vi "Channel plots.vi"(0 "Current time":timestamp[](array[timestamp]), 1 "In Channels":sgl[][](array[numeric]), 3 "Input Channels":dbl[](array[numeric])=[0.0, 0.0, 0.0, 0.0, 0.0, 0.0, 0.0, 0.0, 0.0, 0.0, 0.0, 0.0]) -> (2 "output graph":T1(array[cluster]), 4 "out Ch 1":dbl[](array[numeric]), 5 "out Ch 6":dbl[](array[numeric]), 6 "out Ch 2":dbl[](array[numeric]), 7 "out Ch 3":dbl[](array[numeric]), 8 "out Ch 4":dbl[](array[numeric]), 9 "out Ch 5":dbl[](array[numeric]))   [LabVIEW 2018]
panel:
  # "Ch 0"
  # "Ch 1"
  # "Ch 2"
  # "Ch 3"
  # "Ch 4"
  # "Ch 5"
  # "Ch 6"
  # "Ch 7"
  # "Ch 8"
  # "Ch 9"
  # "Ch 10"
  # "Ch 11"
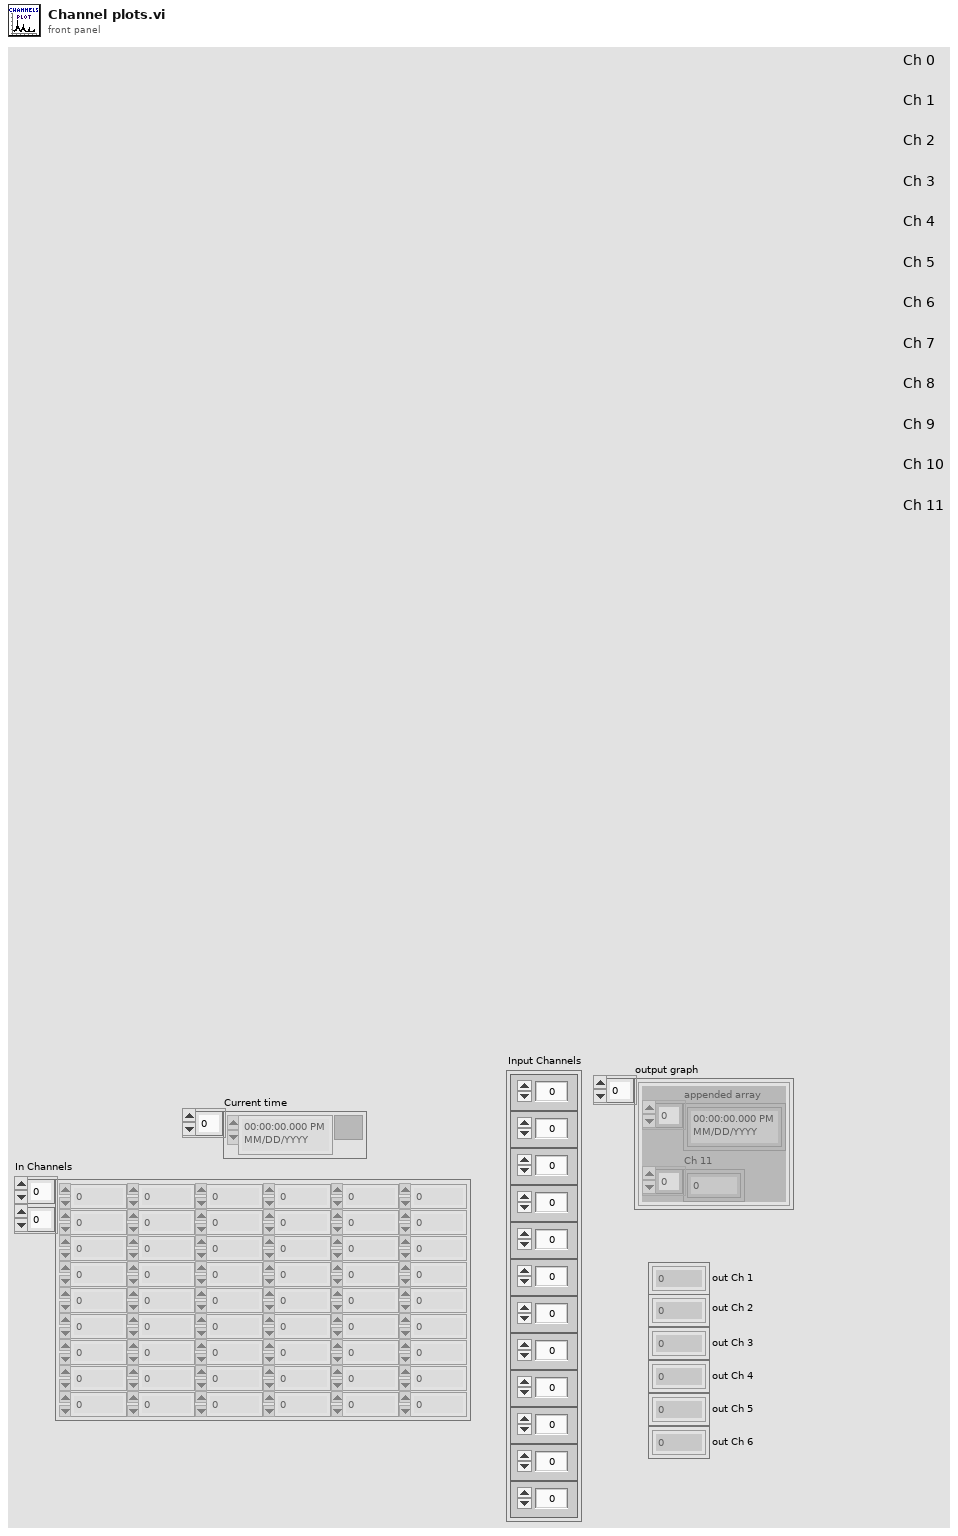
[diagram p1: front panel]
types:
  T1 = cluster{"appended array":timestamp[], "Ch 11":dbl[]}[]
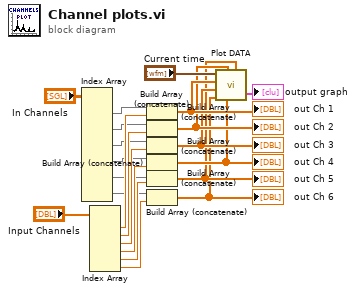
[diagram p0: block diagram]
diagram:
  n1 = Index Array(array="In Channels") -> (element #1=w14:sgl[], element #2=w13:sgl[], element #3=w12:sgl[], element #4=w9:sgl[], element #5=w11:sgl[], element #6=w10:sgl[])  [unwired: 12 in]
  n2 = Index Array(array="Input Channels") -> (element #1=w17:dbl, element #2=w18:dbl, element #3=w19:dbl, element #4=w20:dbl, element #5=w21:dbl, element #6=w22:dbl)  [unwired: 6 in]
  n3 = Build Array (concatenate)(w14, w17) -> (w7:dbl[])
  "out Ch 1" <- w7
  n4 = Build Array (concatenate)(w13, w18) -> (w6:dbl[])
  "out Ch 2" <- w6
  n5 = Build Array (concatenate)(w12, w19) -> (w5:dbl[])
  "out Ch 3" <- w5
  n6 = Build Array (concatenate)(w9, w20) -> (w4:dbl[])
  "out Ch 4" <- w4
  n7 = Build Array (concatenate)(w11, w21) -> (w3:dbl[])
  "out Ch 5" <- w3
  n8 = Build Array (concatenate)(w10, w22) -> (w2:dbl[])
  "out Ch 6" <- w2
  n9 = call "Plot DATA.vi"("Ch 5"=w3, "Ch 4"=w4, "Ch 2"=w6, "Ch 6"=w2, "Ch 3"=w5, "Ch 1"=w7, "Current time"="Current time") -> ("Graph Out"=→"output graph":T1)
